vi "Log-polar transform.vi"(3 "R_min":dbl=10.0, 4 "Log-polar transform size":i32=512, 5 "Complex luminosity gradient map":cdb[][](array[numeric])) -> (0 "drho (y-axis)":dbl, 1 "dtheta (rad, x-axis)":dbl, 2 "Log-polar transform":cdb[][](array[numeric]))   [LabVIEW 2014]
panel:
  # "Paul Nathan 09/06/2015"
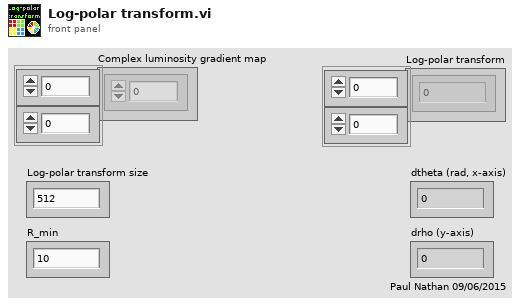
[diagram p1: front panel]
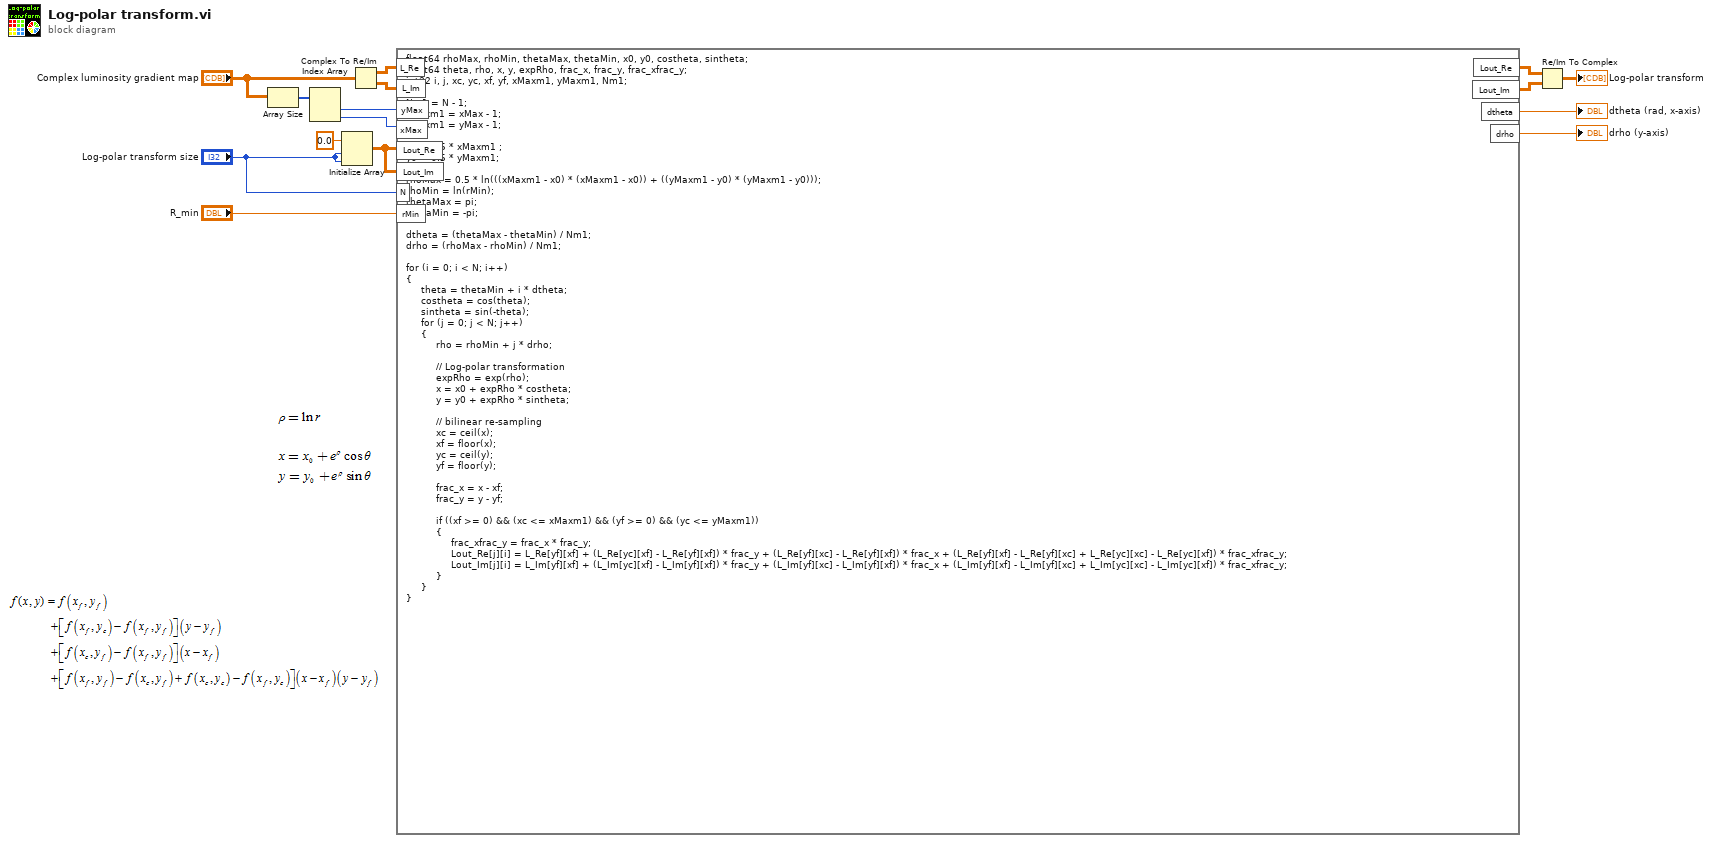
[diagram p0: block diagram]
diagram:
  n1 = Array Size(array="Complex luminosity gradient map") -> (size(s)=w7:i32[])
  n2 = Index Array(array=w7) -> (element #1=w5:i32, element #2=w6:i32)  [unwired: 2 in]
  n3 = Initialize Array(0.0 ("input variable"), "Log-polar transform size", "Log-polar transform size") -> (w13:dbl[][])
  n4 = Complex To Re/Im(x + iy="Complex luminosity gradient map") -> (x=w12:dbl[][], y=w11:dbl[][])
  n5 = formula code="float64 rhoMax, rhoMin, thetaMax, thetaMin, x0, y0, costheta, sintheta;\nfloat64 theta, rho, x, y, expRho, frac_x, frac_y, frac_xfrac_y;\nint32 i, j, xc, yc, xf, yf, xMaxm1, yMaxm1, Nm1;\n\nNm1 = N - 1;\nxMaxm1 = xMax - 1;\nyMaxm1 = yMax - 1;\n\nx0 = 0.5 * xMaxm1 ;\ny0 = 0.5 * yMaxm1; \n\nrhoMax = 0.5 * ln(((xMaxm1 - x0) * (xMaxm1 - x0)) + ((yMaxm1 - y0) * (yMaxm1 - y0)));\nrhoMin = ln(rMin);\nthetaMax = pi;\nthetaMin = -pi;\n\ndtheta = (thetaMax - thetaMin) / Nm1;\ndrho = (rhoMax - rhoMin) / Nm1;\n\nfor (i = 0; i < N; i++)\n{\n     theta = thetaMin + i * dtheta;\n     costheta = cos(theta);\n     sintheta = sin(-theta);\n     for (j = 0; j < N; j++)\n     {\n          rho = rhoMin + j * drho;\n\n          // Log-polar transformation\n          expRho = exp(rho); \n          x = x0 + expRho * costheta;\n          y = y0 + expRho * sintheta;\n          \n          // bilinear re-sampling \n          xc = ceil(x);\n          xf = floor(x);\n          yc = ceil(y);\n          yf = floor(y);\n          \n          frac_x = x - xf;\n          frac_y = y - yf;\n     \n          if ((xf >= 0) && (xc <= xMaxm1) && (yf >= 0) && (yc <= yMaxm1))\n          {\n               frac_xfrac_y = frac_x * frac_y;\n               Lout_Re[j][i] = L_Re[yf][xf] + (L_Re[yc][xf] - L_Re[yf][xf]) * frac_y + (L_Re[yf][xc] - L_Re[yf][xf]) * frac_x + (L_Re[yf][xf] - L_Re[yf][xc] + L_Re[yc][xc] - L_Re[yc][xf]) * frac_xfrac_y;\n               Lout_Im[j][i] = L_Im[yf][xf] + (L_Im[yc][xf] - L_Im[yf][xf]) * frac_y + (L_Im[yf][xc] - L_Im[yf][xf]) * frac_x + (L_Im[yf][xf] - L_Im[yf][xc] + L_Im[yc][xc] - L_Im[yc][xf]) * frac_xfrac_y;     \n          }\n     }\n}"("xMax"=w6, "yMax"=w5, "L_Re"=w12, "Lout_Re"=w13, "rMin"="R_min", "Lout_Im"=w13, "L_Im"=w11, "N"="Log-polar transform size") -> ("Lout_Re"=w10:dbl[][], "dtheta"=→"dtheta (rad, x-axis)":dbl, "drho"=→"drho (y-axis)":dbl, "Lout_Im"=w9:dbl[][])
  n6 = Re/Im To Complex(1:w9, 2:w10) -> (0:→"Log-polar transform":cdb[][])
